vi "ERIO RT STATE Reset Process.vi"(6 "Supervisory Variables In":T4={"Alarm Threshold"=0.0, "Shutdown"=FALSE, "Enable SNS Alarm"=FALSE, "Enable SNS Stage Notification"=FALSE, "Enable SQS Notification"=FALSE, "Enable S3 TDMS Signal Capture"=FALSE, "Enable SystemLink Signal Capture"=FALSE, "Capture Signal"=FALSE, "Server Update"=FALSE, "AWS Access Key"="AKIAINLDO2Y2PDFEWDOQ", "AWS Secret Key"="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", "Phone Number"="+15037066913", "Region"=enum."us-west-2", "AWS SQS Queue"="mynicloud-demotest2", "AWS S3 Bucket"="mynicloud-demotest2"}, 7 "RT State In":T1, 8 "error in (no error)":errorcluster, 9 "AWS Variables In":T6, 11 "EEISysLink.lvclass In":refnum<class "EEISysLink.lvclass">) -> (0 "error out":errorcluster, 1 "AWS Variables Out":T6, 3 "EEISysLink.lvclass Out":refnum<class "EEISysLink.lvclass">, 4 "Supervisory Variables Out":T4={"Alarm Threshold"=0.0, "Shutdown"=FALSE, "Enable SNS Alarm"=FALSE, "Enable SNS Stage Notification"=FALSE, "Enable SQS Notification"=FALSE, "Enable S3 TDMS Signal Capture"=FALSE, "Enable SystemLink Signal Capture"=FALSE, "Capture Signal"=FALSE, "Server Update"=FALSE, "AWS Access Key"="AKIAINLDO2Y2PDFEWDOQ", "AWS Secret Key"="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", "Phone Number"="+15037066913", "Region"=enum."us-west-2", "AWS SQS Queue"="mynicloud-demotest2", "AWS S3 Bucket"="mynicloud-demotest2"}, 5 "RT State Out":T1)   [LabVIEW 2017]
doc: "Reset the simulated conveyor process for another run. The run is driven by encoder position. \n\nJames Tillett P.E.\nEndeavor Engineering Inc.\nwww.endeavoreng.com"
uses:
  Class EEISysLink/EEISysLink.lvclass
  Controls/ERIO AWS Toolkit Variables.ctl
  <vilib>/AWS Toolkit/SQS/Queue/Queue.lvclass
  <vilib>/AWS Toolkit/SNS/Phone Number/Phone Number.lvclass
  <vilib>/AWS Toolkit/S3/Bucket/Bucket.lvclass
  Controls/ERIO Supervisory Variables.ctl
  <vilib>/AWS Toolkit/Core/HTTP Request/Region.ctl
  Controls/ERIO RT State Variables.ctl
  Controls/ERIO SystemStates.ctl
  Controls/ERIO Queue Data.ctl
  Controls/ERIO Worker Variables.ctl
  <vilib>/AWS Toolkit/Core/HTTP Request/HTTP Request.lvclass
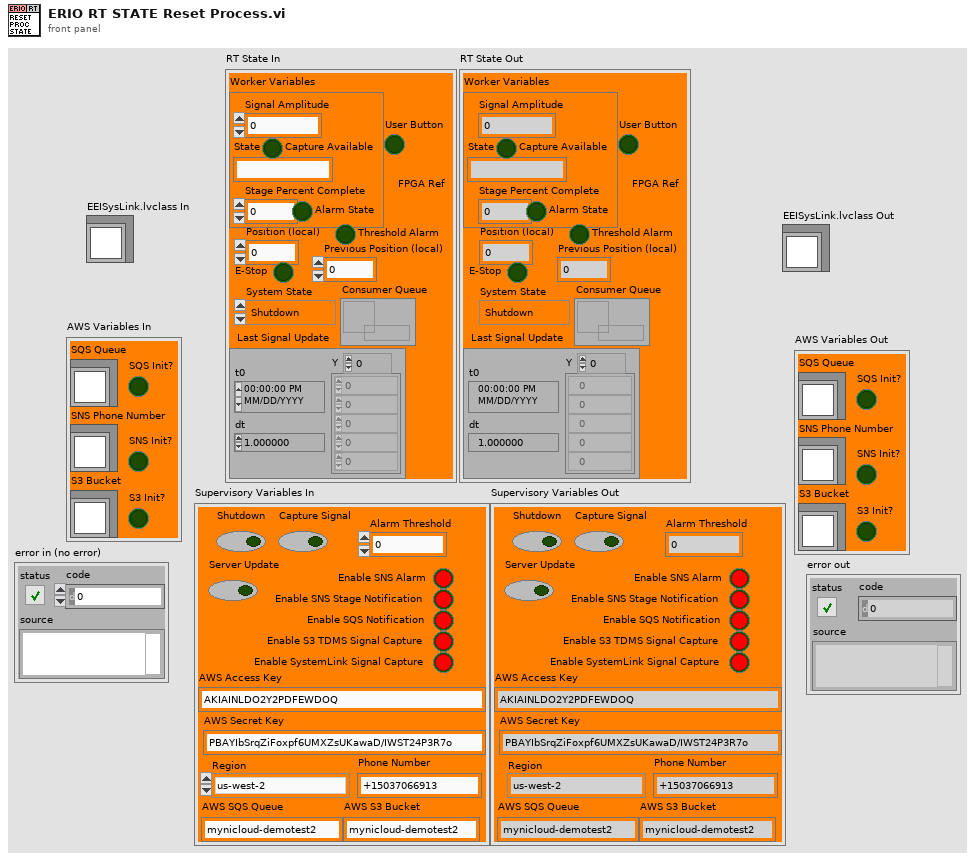
[diagram p1: front panel]
types:
  T1 = typedef "ERIO RT State Variables.ctl" = cluster{"Position (local)":i16, "E-Stop":bool, "System State":T2, "FPGA Ref":refnum<k20>, "Previous Position (local)":i16, "Consumer Queue":refnum<queue>, "Worker Variables":T3, "Threshold Alarm":bool, "User Button":bool, "Last Signal Update":waveform(dbl)}
  T2 = typedef "ERIO SystemStates.ctl" = enum16{"Shutdown", "E-STOP", "Reset Process", "Stage 1", "Stage 2", "Stage 3", "Alarm State"}
  T3 = typedef "ERIO Worker Variables.ctl" = cluster{"Signal Amplitude":dbl, "State":string, "Stage Percent Complete":dbl, "Alarm State":bool, "Capture Available":bool}
  T4 = typedef "ERIO Supervisory Variables.ctl" = cluster{"Alarm Threshold":dbl, "Shutdown":bool, "Enable SNS Alarm":bool, "Enable SNS Stage Notification":bool, "Enable SQS Notification":bool, "Enable S3 TDMS Signal Capture":bool, "Enable SystemLink Signal Capture":bool, "Capture Signal":bool, "Server Update":bool, "AWS Access Key":string, "AWS Secret Key":string, "Phone Number":string, "Region":T5, "AWS SQS Queue":string, "AWS S3 Bucket":string}
  T5 = typedef "NI_AWS_Core.lvlib/HTTP Request.lvclass/Region.ctl" = enum16{"us-east-1", "us-east-2", "us-west-1", "us-west-2", "ap-northeast-1", "ap-northeast-2", "ap-southeast-1", "ap-southeast-2", "ca-central-1", "eu-central-1", "eu-west-1", "eu-west-2", "sa-east-1"}
  T6 = typedef "ERIO AWS Toolkit Variables.ctl" = cluster{"SQS Queue":refnum<class "Queue.lvclass">, "SNS Phone Number":refnum<class "Phone Number.lvclass">, "S3 Bucket":refnum<class "Bucket.lvclass">, "SQS Init?":bool, "S3 Init?":bool, "SNS Init?":bool}
  T7 = typedef "ERIO Queue Data.ctl" = cluster{"Transition Requested":bool, "Current Pos > Previous?":bool, "Amplitude":dbl, "Stage Number":string}
  T8 = typedef "ERIO Stage Transition.ctl" = enum16{"Previous Stage", "Current Stage", "Next Stage"}
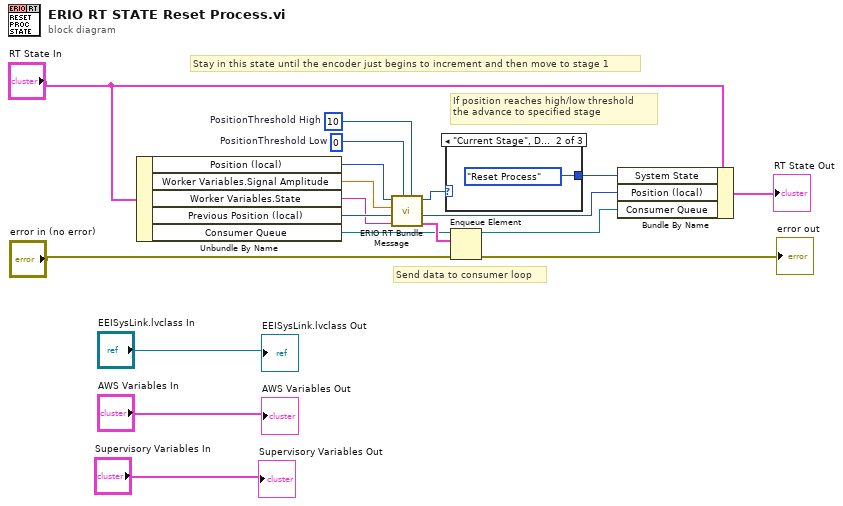
[diagram p0: block diagram]
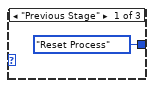
[diagram p2: hidden frame]
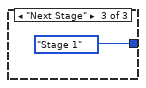
[diagram p3: hidden frame]
diagram:
  w15 = i16 0  # PositionThreshold Low
  w16 = i16 10  # PositionThreshold High
  # "Stay in this state until the encoder just begins to increment and then move to stage 1"
  # "If position reaches high/low threshold \nthe advance to specified stage"
  # "Send data to consumer loop"
  n1 = Unbundle By Name("RT State In") -> ("Position (local)"=w12:i16, "Worker Variables.Signal Amplitude"=w13:dbl, "Worker Variables.State"=w5:string, "Previous Position (local)"=w6:i16, "Consumer Queue"=w9:refnum<queue>)
  n2 = call "ERIO RT Bundle Message.vi"("Position Threshold High"=w16, "Position Threshold Low"=w15, "State"=w5, "Previous Position"=w6, "Amplitude"=w13, "Current Position"=w12) -> ("Output to queue"=w10:T7, "Output Position"=w7:i16, "Transition Action"=w11:T8)  [unwired: 3 in]
  n3 = case shown="\"Current Stage\", Default" w11 {
    tunnel: [ERIO_SystemStates."Reset Process" ("Enum") ERIO_SystemStates."Reset Process" ("Enum") ERIO_SystemStates."Stage 1" ("Enum")] -> w14
    frame "Previous Stage" {
    }
    frame "Current Stage", Default {
    }
    frame "Next Stage" {
    }
  }
  n4 = Enqueue Element(queue=w9, element=w10, error in (no error)="error in (no error)") -> (queue out=w8:refnum<queue>, error out=→"error out":errorcluster)  [unwired: 1 in, 1 out]
  n5 = Bundle By Name(cluster="RT State In", "System State"=w14, "Position (local)"=w7, "Consumer Queue"=w8) -> (→"RT State Out":T1)
  "EEISysLink.lvclass Out" <- "EEISysLink.lvclass In"
  "AWS Variables Out" <- "AWS Variables In"
  "Supervisory Variables Out" <- "Supervisory Variables In"
